vi "TdmsIcons_ReadIcon.vi"(8 "error in (no error)":errorcluster, 10 "Function":string="Add", 11 "TdmsIn":refnum<k34>) -> (0 "error out":errorcluster, 2 "Icon":T1, 3 "TdmsOut":refnum<k34>)   [LabVIEW 2014]
uses:
  <vilib>/picture/picture.llb/imagedata.ctl
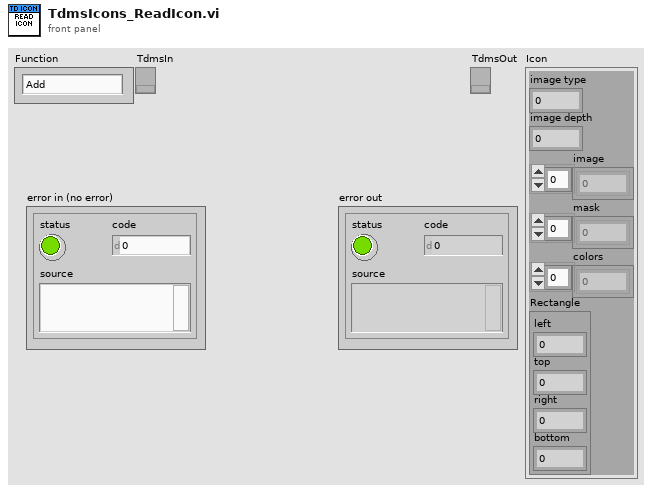
[diagram p1: front panel]
types:
  T1 = typedef "imagedata.ctl" = cluster{"image type":i32, "image depth":i32, "image":u8[], "mask":u8[], "colors":u32[], "Rectangle":cluster{"left":i16, "top":i16, "right":i16, "bottom":i16}}
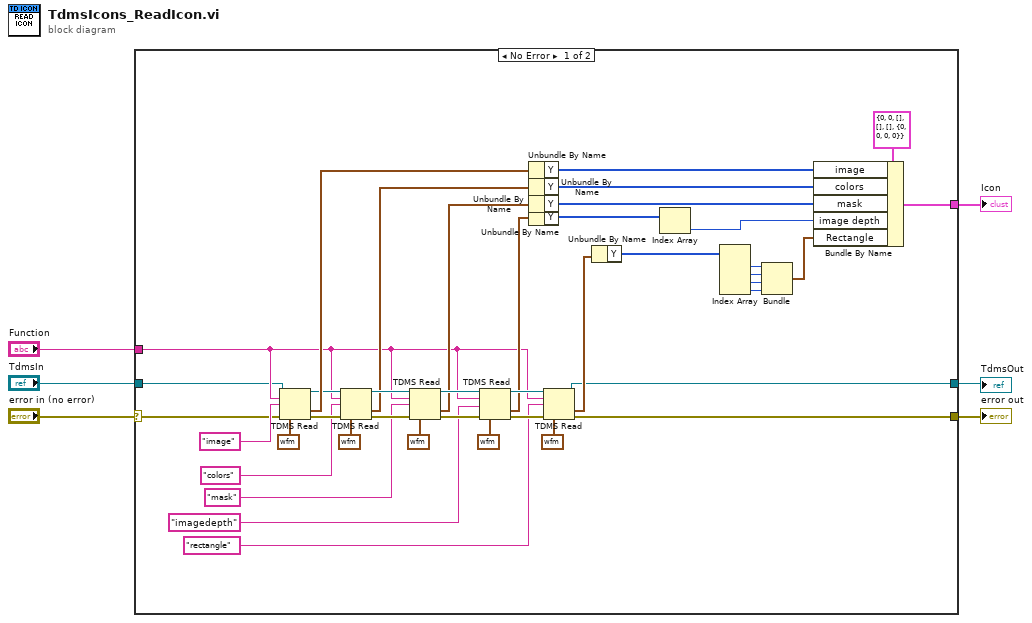
[diagram p0: block diagram]
diagram:
  n1 = case shown="No Error" "error in (no error)" {
    selector: "error in (no error)" -> [w11 w48]
    tunnel: "Function" -> [w19 _]
    tunnel: [w13 w48] -> w5
    tunnel: [w10 w49] -> w4
    tunnel: "TdmsIn" -> [w9 w49]
    tunnel: [w12 _] -> w2
    frame No Error {
      n2 = TDMS Read(0:w9, 5:w19, 7:"image" ("group name in (Untitled)"), 11:w11, 12:waveform(u8) {"t0"=timestamp(0 s since 1904-01-01), "dt"=1.0, "Y"=[]} ("output waveform")) -> (4:w45:refnum<k34>, 10:w47:waveform(u8), 15:w38:errorcluster)  [unwired: 3 in, 3 out]
      n3 = TDMS Read(0:w45, 5:w19, 7:"colors" ("group name in (Untitled)"), 11:w38, 12:waveform(u32) {"t0"=timestamp(0 s since 1904-01-01), "dt"=1.0, "Y"=[]} ("output waveform")) -> (4:w44:refnum<k34>, 10:w37:waveform(u32), 15:w39:errorcluster)  [unwired: 3 in, 3 out]
      n4 = TDMS Read(0:w44, 5:w19, 7:"mask" ("group name in (Untitled)"), 11:w39, 12:waveform(u8) {"t0"=timestamp(0 s since 1904-01-01), "dt"=1.0, "Y"=[]} ("output waveform")) -> (4:w43:refnum<k34>, 10:w36:waveform(u8), 15:w40:errorcluster)  [unwired: 3 in, 3 out]
      n5 = TDMS Read(0:w43, 5:w19, 7:"imagedepth" ("group name in (Untitled)"), 11:w40, 12:waveform(i32) {"t0"=timestamp(0 s since 1904-01-01), "dt"=1.0, "Y"=[]} ("output waveform")) -> (4:w42:refnum<k34>, 10:w35:waveform(i32), 15:w41:errorcluster)  [unwired: 3 in, 3 out]
      n6 = Unbundle By Name(w47) -> ("Y"=w30:u8[])
      n7 = Unbundle By Name(w37) -> ("Y"=w32:u32[])
      n8 = Unbundle By Name(w36) -> ("Y"=w31:u8[])
      n9 = Unbundle By Name(w35) -> ("Y"=w25:i32[])
      n10 = TDMS Read(0:w42, 5:w19, 7:"rectangle" ("group name in (Untitled)"), 11:w41, 12:waveform(i16) {"t0"=timestamp(0 s since 1904-01-01), "dt"=1.0, "Y"=[]} ("output waveform")) -> (4:w10:refnum<k34>, 10:w34:waveform(i16), 15:w13:errorcluster)  [unwired: 3 in, 3 out]
      n11 = Unbundle By Name(w34) -> ("Y"=w29:i16[])
      n12 = Index Array(array=w25) -> (element=w24:i32)  [unwired: 1 in]
      n13 = Index Array(array=w29) -> (element #1=w28:i16, element #2=w27:i16, element #3=w8:i16, element #4=w7:i16)  [unwired: 4 in]
      n14 = Bundle(w28, w27, w8, w7) -> (w26:cluster{i16, i16, i16, i16})  [unwired: 1 in]
      n15 = Bundle By Name(cluster=T1 {"image type"=0, "image depth"=0, "image"=[], "mask"=[], "colors"=[], "Rectangle"={"left"=0, "top"=0, "right"=0, "bottom"=0}} ("Color 256"), "image"=w30, "colors"=w32, "mask"=w31, "image depth"=w24, "Rectangle"=w26) -> (w12:T1)
    }
    frame Error {
    }
  }
  "error out" <- w5
  "TdmsOut" <- w4
  "Icon" <- w2
